vi "Configure Harmonics.vi"(5 "maximum order":i16=1 min=1 max=500 step=1, 7 "minimum order":i8 min=0 max=1 step=1, 8 "error in":errorcluster caption="error in (no error)", 9 "option":u16(ring) items=["ORD", "THD"], 10 "equation":u16(ring) items=["TOT", "FUND"], 11 "VISA resource name":refnum<visa-resource-name>) -> (0 "error out":errorcluster, 3 "VISA resource out":refnum<visa-resource-name>)   [LabVIEW 2018, in "Suita SPAW7000.lvlib"]
uses:
  <instrlib>/Suita SPAW7000/Suita SPAW7000.lvlib
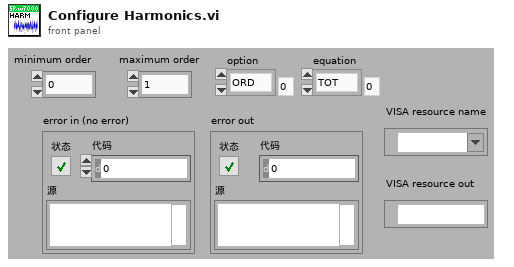
[diagram p1: front panel]
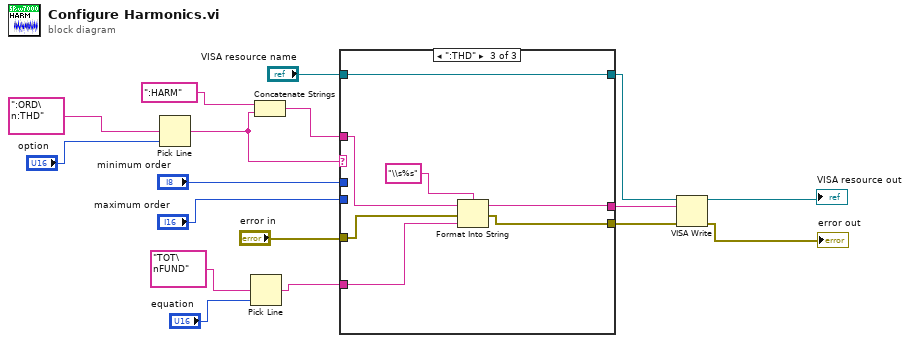
[diagram p0: block diagram]
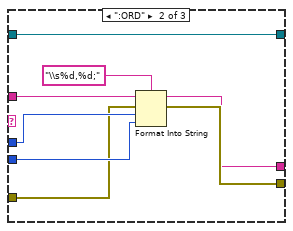
[diagram p3: hidden frame]
diagram:
  n1 = Pick Line(multi-line string=":ORD\n:THD", line index="option") -> (output string=w14:string)  [unwired: 1 in]
  n2 = Pick Line(multi-line string="TOT\nFUND", line index="equation") -> (output string=w8:string)  [unwired: 1 in]
  n3 = Concatenate Strings(":HARM", w14) -> (w11:string)
  n4 = case shown="\":THD\"" w14 {
    tunnel: "minimum order" -> [_ w28 _]
    tunnel: "maximum order" -> [_ w27 _]
    tunnel: w11 -> [w19 w26 w34]
    tunnel: "error in" -> [w20 w24 w31]
    tunnel: [w20 w23 w30] -> w7
    tunnel: [w19 w22 w32] -> w6
    tunnel: w8 -> [_ _ w35]
    tunnel: "VISA resource name" -> [w18 w21 w29]
    tunnel: [w18 w21 w29] -> w4
    frame Default {
    }
    frame ":ORD" {
      n5 = Format Into String(format string="\\s%d,%d;" ("格式字符串"), initial string=w26, error in=w24, w28, w27) -> (resulting string=w22:string, error out=w23:errorcluster)
    }
    frame ":THD" {
      n6 = Format Into String(format string="\\s%s" ("格式字符串"), initial string=w34, error in=w31, w35) -> (resulting string=w32:string, error out=w30:errorcluster)
    }
  }
  n7 = VISA Write(VISA resource name=w4, write buffer=w6, error in (no error)=w7) -> (VISA resource name out=→"VISA resource out":refnum<visa-resource-name>, error out=→"error out":errorcluster)  [unwired: 1 out]
